vi "maszynas stanow do arduino.vi"() -> ()   [LabVIEW 2026]
doc: "Use this template to build a standard state machine design pattern. Each state executes code and determines which state to transition to. Contrast this design pattern with the User Interface Event Handler pattern, in which code executes in response to user actions. Contrast this design pattern also with the Queued Message Handler pattern, in which each message handling code can queue zero or more new messages.\nNote: This template does not contain the most recent programming guidelines recommended by National Instruments. For a complete, project-based implementation of the Standard State Machine pattern, use the Create Project dialog box instead of this template."
uses:
  <vilib>/MakerHub/LINX/Private/Type Defs/LINX Ref.ctl
  <vilib>/MakerHub/LINX/Private/Type Defs/Platform.ctl
  <vilib>/MakerHub/LINX/Private/Type Defs/Interface.ctl
  <vilib>/MakerHub/LINX/Private/Device/Type Defs/LINX Device Config.ctl
  <vilib>/MakerHub/LINX/Private/Device/Type Defs/TCP Config.ctl
  <vilib>/MakerHub/LINX/Private/Device/Type Defs/Channels.ctl
  maszynas stanow do arudino.ctl
  <vilib>/MakerHub/LINX/Public/Utilities/Open Local.vi
  <vilib>/MakerHub/LINX/LMH-LINX.lvlib
  <vilib>/MakerHub/LINX/Private/Device/Device.lvlib
panel:
  out "Error Out":errorcluster
  out "Array":i32[](array[numeric])
  in  "LINX Resource":T1
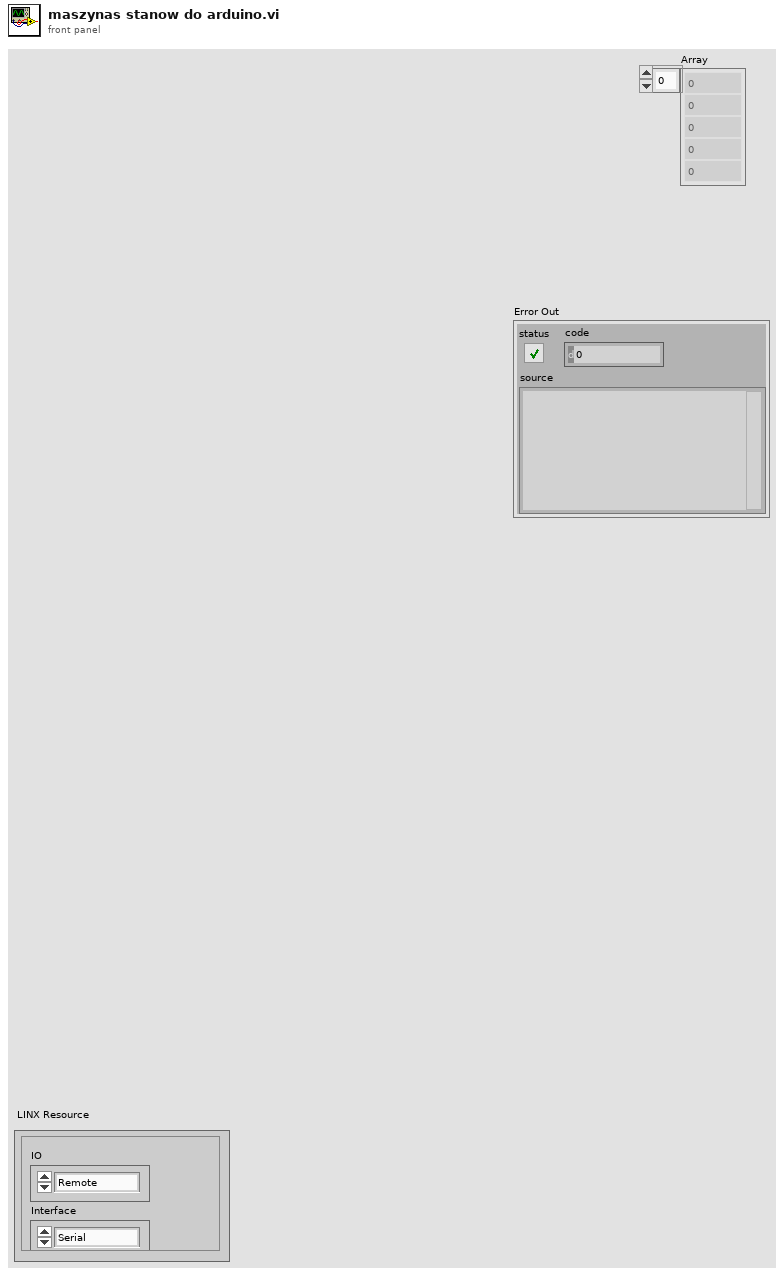
[diagram p1: front panel]
types:
  T1 = typedef "LMH-LINX.lvlib/LINX Ref.ctl" = cluster{"IO":T2, "Interface":T3, "LINX Device Config":T4}
  T2 = typedef "LMH-LINX.lvlib/Platform.ctl" = enum16{"Remote", "Local"}
  T3 = typedef "LMH-LINX.lvlib/Interface.ctl" = enum16{"Serial", "TCP"}
  T4 = typedef "LMH-LINX.lvlib/Device.lvlib/LINX Device Config.ctl" = cluster{"Interface":T3, "COM Port":refnum<visa-resource-name>, "TCP Configuration":T5, "Device Family":u8, "Device ID":u8, "Device Name":string, "TCP Ref":refnum<k5>, "Channels":T6}
  T5 = typedef "LMH-LINX.lvlib/Device.lvlib/TCP Config.ctl" = cluster{"IP Address":string, "Port":u16}
  T6 = typedef "LMH-LINX.lvlib/Channels.ctl" = cluster{"DI":u8[], "DO":u8[], "AI":u8[], "AO":u8[], "PWM":u8[], "QE":u8[], "UART":u8[], "I2C 2":u8[], "SPI":u8[], "CAN":u8[], "Servo":u8[], "AI Ref (V)":dbl, "AI Resolution (Bits)":u8, "AO Ref (V)":dbl, "AO Resolution (Bits)":u8}
  T7 = typedef "maszynas stanow do arudino.ctl" = enum16{"Set by py", "Initialize", "Stop"}
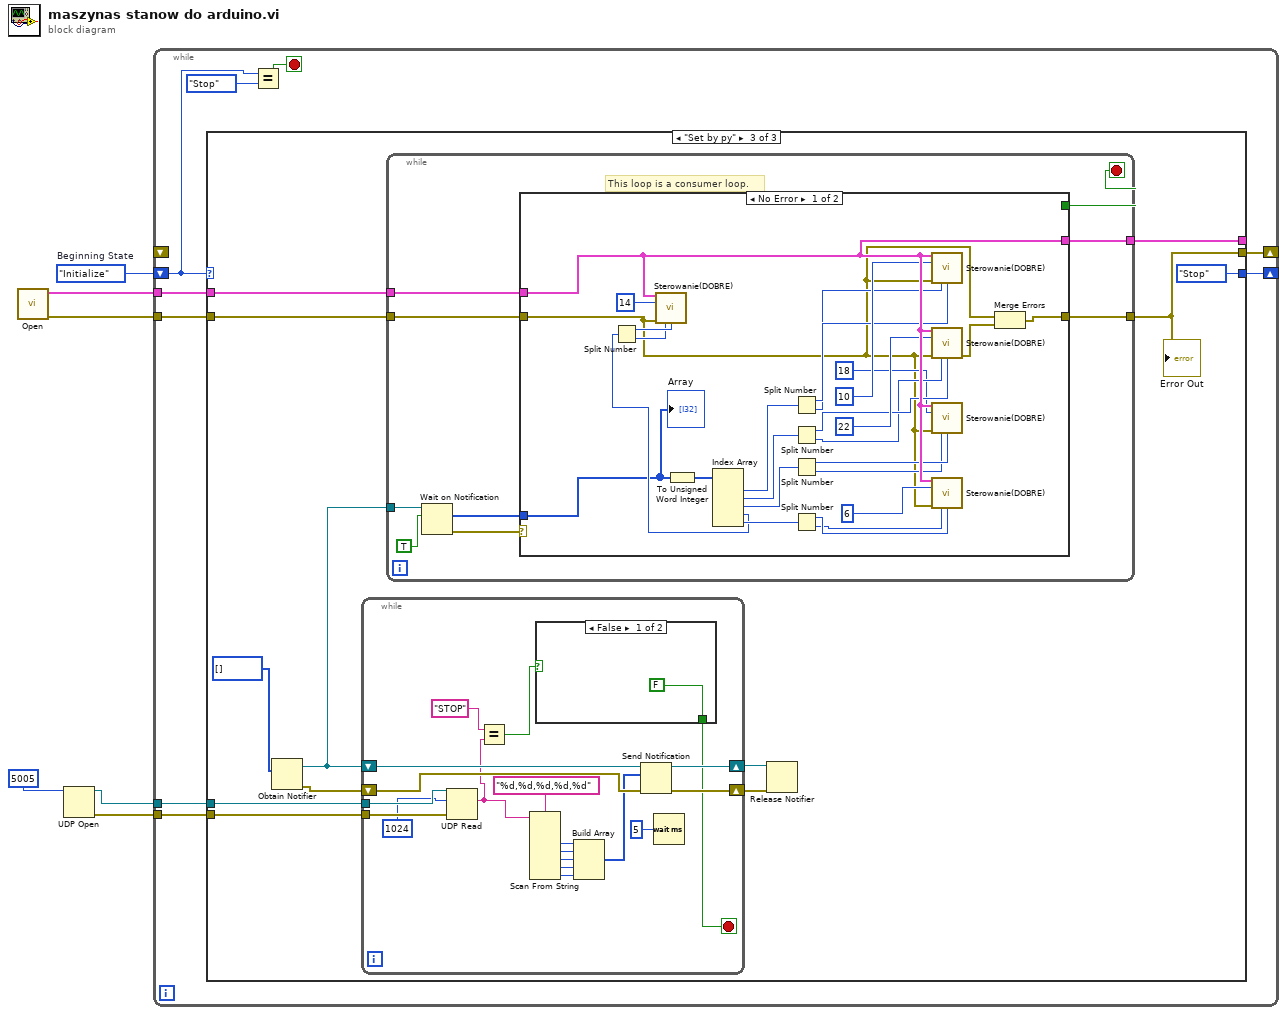
[diagram p0: block diagram]
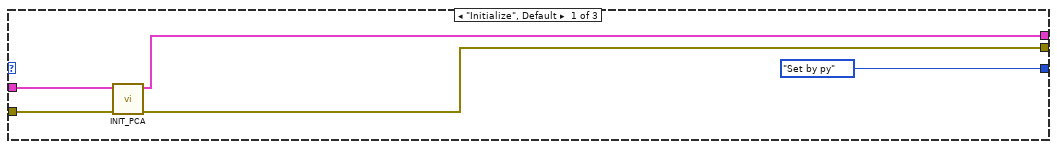
[diagram p2: hidden frame]
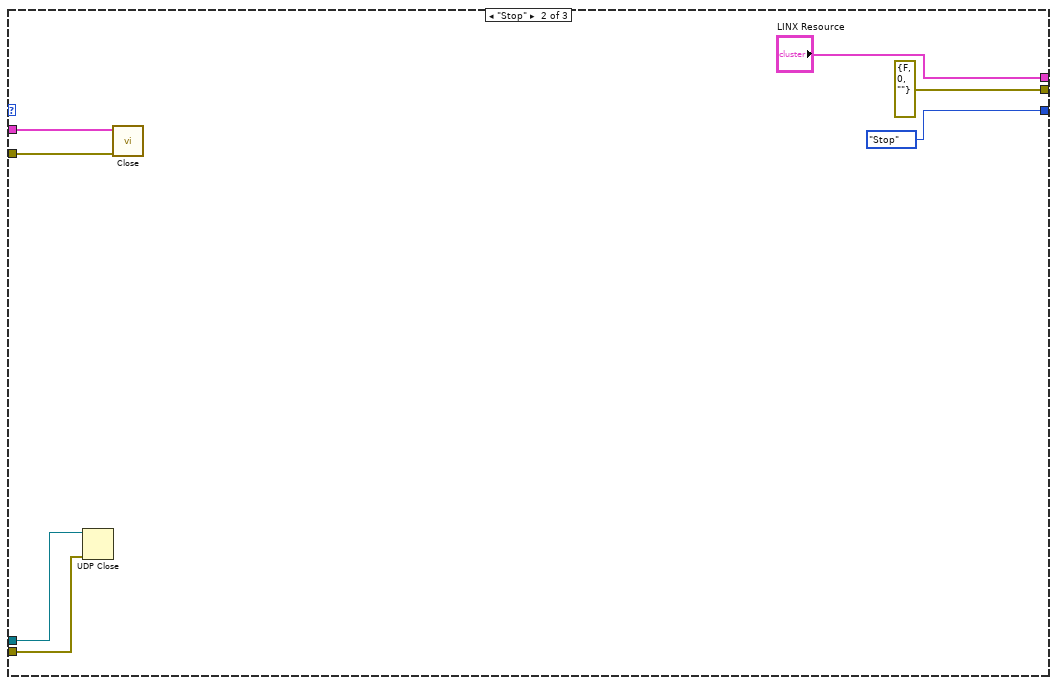
[diagram p3: hidden frame]
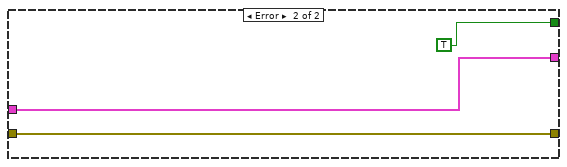
[diagram p4: hidden frame]
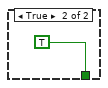
[diagram p5: hidden frame]
diagram:
  w6 = maszynas_stanow_do_arudino."Initialize"  # Beginning State
  n1 = call-poly <vilib>:"Open.vi"() -> ("Error Out"=w4:errorcluster, "LINX Resource"=w5:T1)  [unwired: 9 in, 1 out]
  n2 = UDP Open(11:u16 5005 ("port")) -> (port=w2:refnum<k16>, 0:w1:errorcluster)  [unwired: 4 in, 1 out]
  n3 = while {
    shift-right: [w13] -> _
    shift-left: w6 -> [w10]
    tunnel: w5 -> [w12]
    tunnel: w4 -> [w9]
    shift-right: [w11] -> _
    shift-left: _ -> [_]
    tunnel: w2 -> [w8]
    tunnel: w1 -> [w7]
    stop <- w15 stop-if-true
    n4 = case shown="\"Set by py\"" w10 {
      tunnel: [maszynas_stanow_do_arudino."Set by py" ("States") maszynas_stanow_do_arudino."Stop" ("Next State") maszynas_stanow_do_arudino."Stop" ("States")] -> w13
      tunnel: w12 -> [w19 w24 w37]
      tunnel: w9 -> [w18 w23 w32]
      tunnel: [w17 "LINX Resource" w38] -> _
      tunnel: [w16 errorcluster {"status"=FALSE, "code"=0, "source"=""} ("Error Out") w28] -> w11
      tunnel: w8 -> [_ w22 w31]
      tunnel: w7 -> [_ w21 w30]
      frame "Initialize", Default {
        n5 = call "INIT_PCA.vi"("Error In"=w18, "LINX Resource 2"=w19) -> ("error out"=w16:errorcluster, "LINX Resource"=w17:T1)  [unwired: 8 in]
      }
      frame "Stop" {
        n6 = UDP Close(connection ID=w22, 8:w21) -> ()  [unwired: 2 out]
        n7 = call <vilib>:"Close.vi"("Error In"=w23, "LINX Resource"=w24) -> ()  [unwired: 9 in, 1 out]
      }
      frame "Set by py" {
        n8 = Obtain Notifier(notification data type=i32[] []) -> (notifier out=w35:refnum<notifier>, error out=w29:errorcluster)  [unwired: 3 in, 1 out]
        n9 = while {
          shift-right: [w94] -> w33
          shift-left: w29 -> [w95]
          shift-right: [w93] -> w34
          shift-left: w35 -> [w92]
          tunnel: w31 -> [w91]
          tunnel: w30 -> [w90]
          stop <- w78 stop-if-true
          n10 = UDP Read(connection ID=w91, max size (548)=1024, 8:w90) -> (data out=w81:string)  [unwired: 1 in, 4 out]
          n11 = Equal?(x="STOP", y=w81) -> (x = y?=w79:bool)
          n12 = Scan From String(format string="%d,%d,%d,%d,%d", input string=w81) -> (output 1=w87:i32, output 2=w86:i32, output 3=w85:i32, output 4=w84:i32, output 5=w83:i32)  [unwired: 7 in, 3 out]
          n13 = case shown="False" w79 {
            tunnel: [FALSE TRUE] -> w78
            frame False {
            }
            frame True {
            }
          }
          n14 = Build Array(w87, w86, w85, w84, w83) -> (w82:i32[])
          n15 = Send Notification(notification=w82, notifier=w92, error in (no error)=w95) -> (notifier out=w93:refnum<notifier>, error out=w94:errorcluster)
          n16 = Wait (ms)(milliseconds to wait=u32 5) -> ()  [unwired: 1 out]
        }
        n17 = while {
          tunnel: w35 -> [w44]
          tunnel: w37 -> [w47]
          tunnel: [w46] -> w28
          tunnel: [w45] -> w38
          tunnel: w32 -> [w40]
          stop <- w48 stop-if-true
          # "This loop is a consumer loop."
          n18 = Wait on Notification(notifier=w44, ignore previous (F)=TRUE) -> (notification=w43:i32[], error out=w41:errorcluster)  [unwired: 2 in, 2 out]
          n19 = case shown="No Error" w41 {
            tunnel: [_ TRUE] -> w48
            tunnel: w47 -> [w73 w76]
            tunnel: w40 -> [w52 w75]
            tunnel: [w50 w75] -> w46
            tunnel: [w73 w76] -> w45
            tunnel: w43 -> [w49 _]
            frame No Error {
              n20 = To Unsigned Word Integer(number=w49) -> (unsigned 16bit integer=w74:u16[])
              n21 = Index Array(array=w74) -> (element #1=w53:u16, element #2=w72:u16, element #3=w71:u16, element #4=w54:u16, element #5=w70:u16)  [unwired: 5 in]
              n22 = Split Number(x=w54) -> (hi(x)=w56:u8, lo(x)=w55:u8)
              n23 = call "Sterowanie(DOBRE).vi"("LINX Resource in"=w73, "element"=u8 14, "error in (no error)"=w52, "element 4"=w55, "element 5"=w56) -> ()  [unwired: 9 in, 2 out]
              n24 = Split Number(x=w53) -> (hi(x)=w68:u8, lo(x)=w67:u8)
              n25 = Split Number(x=w72) -> (hi(x)=w65:u8, lo(x)=w64:u8)
              n26 = Split Number(x=w71) -> (hi(x)=w62:u8, lo(x)=w61:u8)
              n27 = Split Number(x=w70) -> (hi(x)=w59:u8, lo(x)=w58:u8)
              n28 = call "Sterowanie(DOBRE).vi"("LINX Resource in"=w73, "element"=u8 10, "error in (no error)"=w52, "element 4"=w67, "element 5"=w68) -> ()  [unwired: 9 in, 2 out]
              n29 = call "Sterowanie(DOBRE).vi"("LINX Resource in"=w73, "element"=u8 22, "error in (no error)"=w52, "element 4"=w64, "element 5"=w65) -> ("error out"=w51:errorcluster)  [unwired: 9 in, 1 out]
              n30 = call "Sterowanie(DOBRE).vi"("LINX Resource in"=w73, "element"=u8 18, "error in (no error)"=w52, "element 4"=w61, "element 5"=w62) -> ()  [unwired: 9 in, 2 out]
              n31 = call "Sterowanie(DOBRE).vi"("LINX Resource in"=w73, "element"=u8 6, "error in (no error)"=w52, "element 4"=w58, "element 5"=w59) -> ()  [unwired: 9 in, 2 out]
              n32 = Merge Errors(w52, w51) -> (w50:errorcluster)
              "Array" <- w49
            }
            frame Error {
            }
          }
        }
        "Error Out" <- w28
        n33 = Release Notifier(notifier=w34, error in (no error)=w33) -> ()  [unwired: 1 in, 3 out]
      }
    }
    n34 = Equal?(x=w10, y=maszynas_stanow_do_arudino."Stop" ("States")) -> (x = y?=w15:bool)
  }
